vi "Video Stuff v01.vi"() -> ()   [LabVIEW 2009]
doc: "The Grab and Select Mode VI acquires images continuously and displays the images in an image control using high-level acquisition VIs. This example also demonstrates the capability to enumerate and change the video mode. A grab is appropriate for high-speed applications in which you need to process only one image at a time. This example requires a FireWire camera."
uses:
  <vilib>/userDefined/High Color/IMAQdx.ctl
  <vilib>/vision/driver/NI_Vision_Acquisition_Software.lvlib
  Program Files/National Instruments/LabVIEW 2009/resource/objmgr/imaqdx.rc
  <vilib>/vision/NI_Vision_Development_Module.lvlib
panel:
  out "Teh X4m":T1(plugin-control)
  in  "Interpolation Type":u32(ring) items=["Zero Order", "Bi-Linear", "Quadratic", "Cubic Spline"]
  out "Calibrated Image":T1(plugin-control)
  in  "Grid Descriptor":T2={"X Step"=1.0, "Y Step"=1.0, "Unit"=enum."Undefined", "Threshold Range"={"Lower value"=30.0, "Upper value"=96.0}} {"Threshold Range"."Upper value" format="%.2f"; "Threshold Range"."Lower value" format="%.2f"; "Y Step" format="%.2f"; "X Step" format="%.2f"}
  in  "Calibration Learn Setup":T4={"Distortion"=0, "Corrected Image Scaling"=0, "Corrected Image Learn ROI"=2, "Learn Error Map?"=FALSE, "Learn Correction Table?"=FALSE} {"Corrected Image Learn ROI" items=["Full Image ", "Calibration ROI", "ROI", "Calibration AND ROI", "Calibration OR ROI"]; "Corrected Image Scaling" items=["Scale to Preserve Area", "Scale to Fit"]; "Distortion" items=["Perspective", "Nonlinear"]}
  out "Calibration Image":T1(plugin-control)
  out "Super Filter":T1(plugin-control)
  in  "Red Range":cluster{"Lower value":i32, "Upper value":i32}={"Lower value"=240, "Upper value"=255}
  in  "Green Range":cluster{"Lower value":i32, "Upper value":i32}={"Lower value"=250, "Upper value"=255}
  in  "Blue Range":cluster{"Lower value":i32, "Upper value":i32}={"Lower value"=250, "Upper value"=255}
  in  "Color Mode":u16(ring) items=["RGB", "HSL", "HSV", "HSI"]
  out "Frame Rate":dbl(knob) scale=0.0..100.0 scale format="%.1f"
  in  "Camera Name":T5
  out "Buffer Number":u32
  out "Image":T1(plugin-control)
  in  "stop":bool
  in  "Video Modes":i32(listbox)
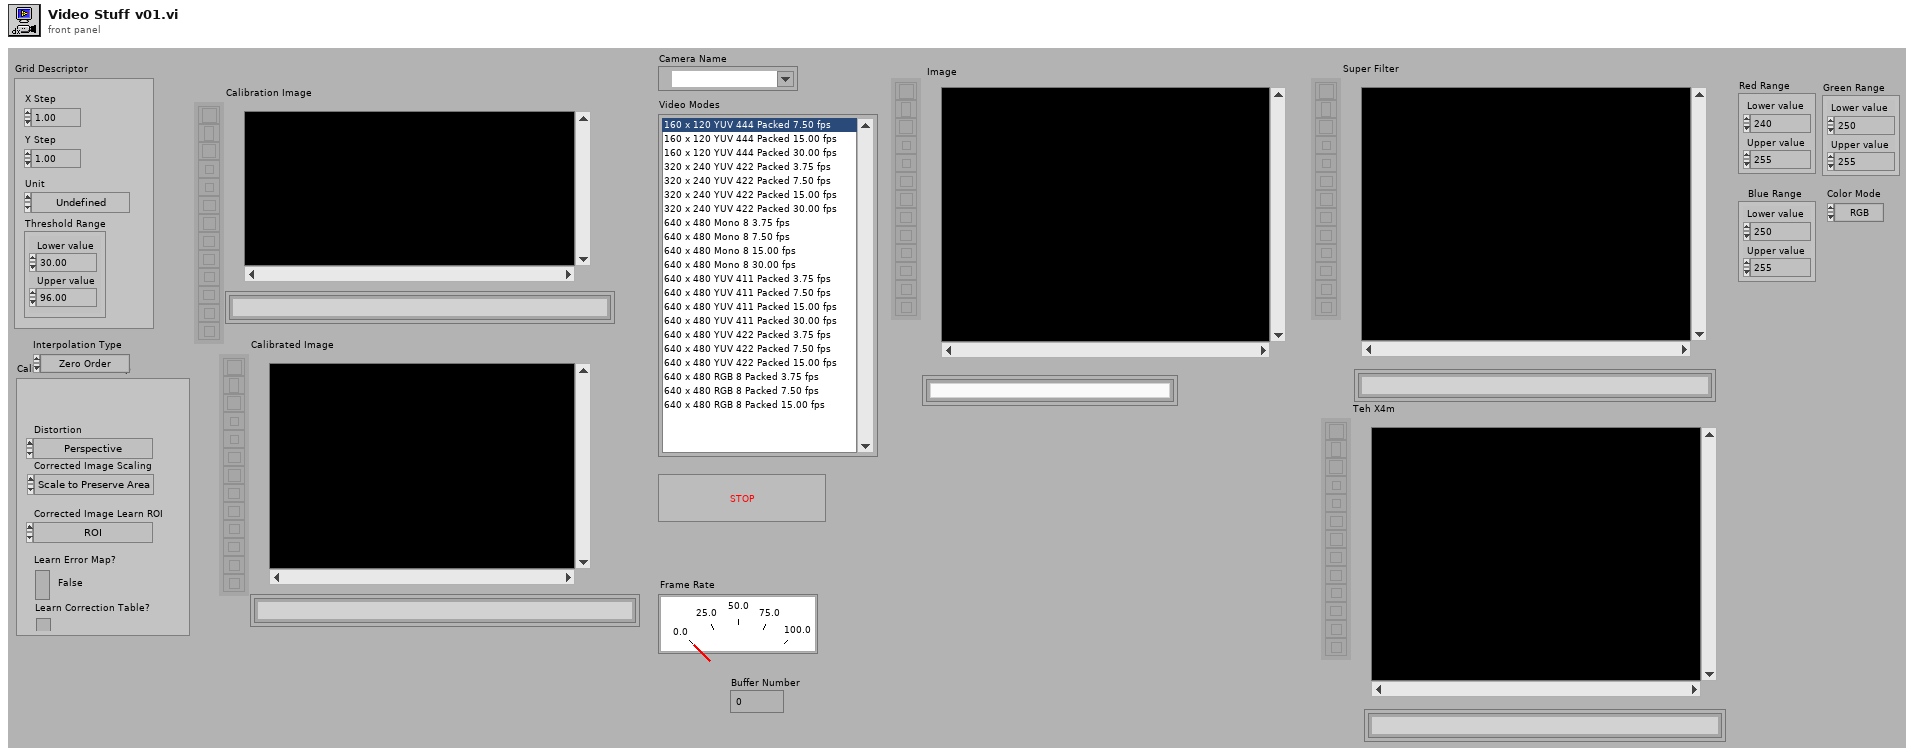
[diagram p1: front panel]
types:
  T1 = typedef "IMAQ Image.ctl" = refnum<image>
  T2 = typedef "Grid Descriptor" = cluster{"X Step":sgl, "Y Step":sgl, "Unit":T3, "Threshold Range":cluster{"Lower value":sgl, "Upper value":sgl}}
  T3 = typedef "Image Unit" = enum32{"Undefined", "Angström", "Micrometer", "Millimeter", "Centimeter", "Meter", "Kilometer", "Microinch", "Inch", "Feet", "Nautical miles", "Standard miles", "Steps"}
  T4 = cluster{"Distortion":u32, "Corrected Image Scaling":u32, "Corrected Image Learn ROI":u32, "Learn Error Map?":bool, "Learn Correction Table?":bool}
  T5 = typedef "IMAQdx.ctl" = refnum<k21>
  T6 = typedef "Image Type" = u32
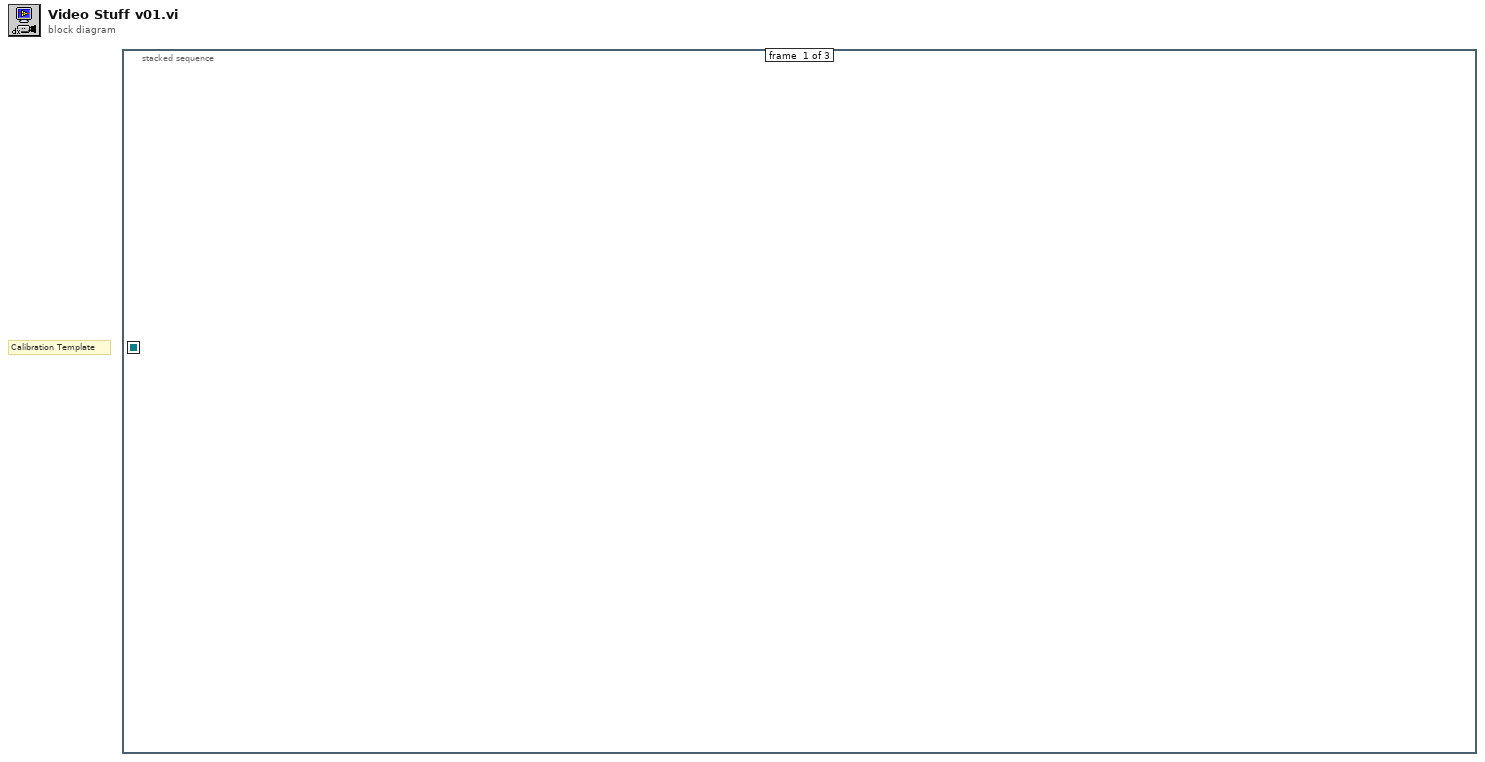
[diagram p0: block diagram]
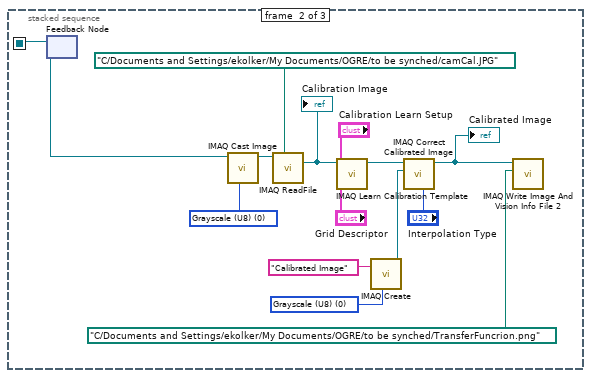
[diagram p2: hidden frame]
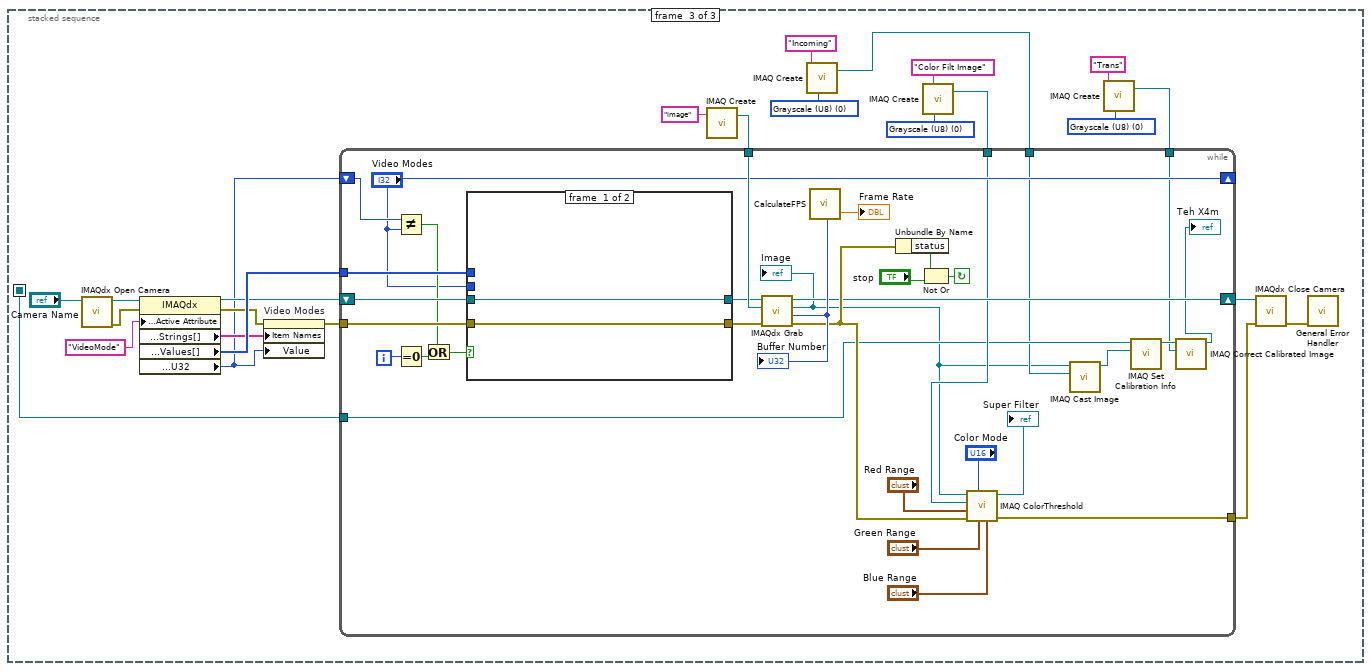
[diagram p3: hidden frame]
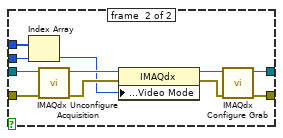
[diagram p4: hidden frame]
diagram:
  # "Calibration Template"
  n1 = stacked-sequence {
    seq-local: [_ w1 _] -> [_ _ w22]
    frame #0 {
    }
    frame #1 {
      w6 = T6 0 items=["Grayscale (U8)", "Grayscale (I16)", "Grayscale (SGL)", "Complex (CSG)", "RGB (U32)", "HSL (U32)", "RGB (U64)", "Grayscale (U16)"] ("Image Type")
      w15 = T6 0 items=["Grayscale (U8)", "Grayscale (I16)", "Grayscale (SGL)", "Complex (CSG)", "RGB (U32)", "HSL (U32)", "RGB (U64)", "Grayscale (U16)"] ("Image Type")
      n2 = feedback #1() -> (w1:T1)  [unwired: 1 in]
      n3 = call "IMAQ Cast Image"("Image Type"=w6, "Image Src"=w1) -> ("Image Dst Out"=w7:T1)  [unwired: 8 in, 1 out]
      n4 = call "IMAQ ReadFile"("File Path"=path "C:/Documents and Settings/ekolker/My Documents/OGRE/to be synched/camCal.JPG" ("Calibration Image"), "Image"=w7) -> ("Image Out"=w13:T1)  [unwired: 5 in, 4 out]
      "Calibration Image" <- w13
      n5 = call "IMAQ Learn Calibration Template"("Grid Descriptor"="Grid Descriptor", "Calibration Learn Setup"="Calibration Learn Setup", "Image"=w13) -> ("Calibrated Image"=w10:T1)  [unwired: 6 in, 2 out]
      n6 = call "IMAQ Create"("Image Name"="Calibrated Image", "Image Type"=w15) -> ("New Image"=w9:T1)  [unwired: 2 in, 2 out]
      n7 = call "IMAQ Correct Calibrated Image"("Interpolation Type"="Interpolation Type", "Image Dst"=w9, "Image Src"=w10) -> ("Corrected Image"=w4:T1)  [unwired: 7 in, 1 out]
      "Calibrated Image" <- w4
      n8 = call "IMAQ Write Image And Vision Info File 2"("File Path"=path "C:/Documents and Settings/ekolker/My Documents/OGRE/to be synched/TransferFuncrion.png" ("Calibration\nData File"), "Image"=w4) -> ("Image Out (duplicate)"=w2:T1)  [unwired: 8 in, 1 out]
    }
    frame #2 {
      w17 = T6 0 items=["Grayscale (U8)", "Grayscale (I16)", "Grayscale (SGL)", "Complex (CSG)", "RGB (U32)", "HSL (U32)", "RGB (U64)", "Grayscale (U16)"] ("Image Type")
      w20 = T6 0 items=["Grayscale (U8)", "Grayscale (I16)", "Grayscale (SGL)", "Complex (CSG)", "RGB (U32)", "HSL (U32)", "RGB (U64)", "Grayscale (U16)"] ("Image Type")
      w24 = T6 0 items=["Grayscale (U8)", "Grayscale (I16)", "Grayscale (SGL)", "Complex (CSG)", "RGB (U32)", "HSL (U32)", "RGB (U64)", "Grayscale (U16)"] ("Image Type")
      n9 = call <vilib>:"IMAQdx Open Camera.vi"("Session In"="Camera Name") -> ("error out"=w33:errorcluster, "Session Out"=w36:T5)  [unwired: 2 in, 7 out]
      n10 = property class="IMAQdx"(reference=w36, error in=w33, "Camera Attributes:Active Attribute"="VideoMode" ("ActiveAttribute")) -> (reference out=w31:T5, error out=w32:errorcluster, "Camera Attributes:Enum:Strings[]"=w29:string[], "Camera Attributes:Enum:Values[]"=w34:u32[], "Camera Attributes:Value:U32"=w28:u32)
      n11 = property on="Video Modes" class="ListBox (strict)"(error in=w32, "Item Names"=w29, "Value"=w28) -> (error out=w30:errorcluster)  [unwired: 1 in, 1 out]
      n12 = call "IMAQ Create"("Image Name"="image") -> ("New Image"=w39:T1)  [unwired: 3 in, 2 out]
      n13 = call "IMAQ Create"("Image Name"="Incoming", "Image Type"=w17) -> ("New Image"=w16:T1)  [unwired: 2 in, 2 out]
      n14 = call "IMAQ Create"("Image Name"="Color Filt Image", "Image Type"=w24) -> ("New Image"=w25:T1)  [unwired: 2 in, 2 out]
      n15 = call "IMAQ Create"("Image Name"="Trans", "Image Type"=w20) -> ("New Image"=w19:T1)  [unwired: 2 in, 2 out]
      n16 = while {
        tunnel: w34 -> [w70]
        shift-left: w28 -> [w58]
        shift-right: ["Video Modes"] -> _
        tunnel: w39 -> [w71]
        tunnel: w30 -> [w72]
        shift-right: [w51] -> w38
        shift-left: w31 -> [w73]
        tunnel: w25 -> [w50]
        tunnel: [w49] -> w23
        tunnel: w22 -> [w46]
        tunnel: w19 -> [w45]
        tunnel: w16 -> [w44]
        i -> [w64]
        stop <- w67 continue-if-true
        n17 = Not Equal?(x=w58, y="Video Modes") -> (x != y?=w65:bool)
        n18 = Equal To 0?(x=w64) -> (x = 0?=w63:bool)
        n19 = Or(x=w65, y=w63) -> (x .or. y?=w66:bool)
        n20 = case shown="True" w66 {
          tunnel: w73 -> [w75 w84]
          tunnel: w72 -> [w74 w83]
          tunnel: [w75 w80] -> w61
          tunnel: [w74 w81] -> w62
          tunnel: w70 -> [_ w86]
          tunnel: "Video Modes" -> [_ w85]
          frame #0 {
          }
          frame #1 {
            n21 = Index Array(array=w86, index=w85) -> (element=w76:u32)
            n22 = call <vilib>:"IMAQdx Unconfigure Acquisition.vi"("error in"=w83, "Session In"=w84) -> ("error out"=w77:errorcluster, "Session Out"=w82:T5)  [unwired: 8 out]
            n23 = property class="IMAQdx"(reference=w82, error in=w77, "Acquisition Attributes:Video Mode"=w76) -> (reference out=w79:T5, error out=w78:errorcluster)
            n24 = call <vilib>:"IMAQdx Configure Grab.vi"("error in"=w78, "Session In"=w79) -> ("error out"=w81:errorcluster, "Session Out"=w80:T5)  [unwired: 1 in, 7 out]
          }
        }
        n25 = call <vilib>:"IMAQdx Grab.vi"("error in"=w62, "Image In"=w71, "Session In"=w61) -> ("error out"=w56:errorcluster, "Buffer Number Out"=w59:u32, "Image Out"=w43:T1, "Session Out"=w51:T5)  [unwired: 1 in, 4 out]
        "Image" <- w43
        "Buffer Number" <- w59
        n26 = call "CalculateFPS.vi"("buffer number"=w59) -> ("processed FPS"=→"Frame Rate":dbl)  [unwired: 2 out]
        n27 = Unbundle By Name(w56) -> ("status"=w68:bool)
        n28 = Not Or(1:"stop", 2:w68) -> (0:w67:bool)
        n29 = call "IMAQ ColorThreshold"("Blue or Luma or Val or Inten Range"="Blue Range", "Green or Sat Range"="Green Range", "Color Mode"="Color Mode", "error in (no error)"=w56, "Red or Hue Range"="Red Range", "Image Dst"=w50, "Image Src"=w43) -> ("error out"=w49:errorcluster, "Image Dst Out"=→"Super Filter":T1)  [unwired: 3 in]
        n30 = call "IMAQ Cast Image"("Image Dst"=w44, "Image Src"=w43) -> ("Image Dst Out"=w42:T1)  [unwired: 8 in, 1 out]
        n31 = call "IMAQ Set Calibration Info"("Image Dst"=w42, "Image Src"=w46) -> ("Calibrated Image"=w47:T1)  [unwired: 2 in, 7 out]
        n32 = call "IMAQ Correct Calibrated Image"("Image Dst"=w45, "Image Src"=w47) -> ("Corrected Image"=→"Teh X4m":T1)  [unwired: 5 in, 4 out]
      }
      n33 = call <vilib>:"IMAQdx Close Camera.vi"("error in"=w23, "Session In"=w38) -> ("error out"=w27:errorcluster)  [unwired: 9 out]
      n34 = call <vilib>:"General Error Handler.vi"("error in (no error)"=w27) -> ()  [unwired: 1 in, 14 out]
    }
  }
